vi "CANOpen_SetGet NMT Settings.vi"(6 "Set Parameters":bool, 8 "error in (no error)":errorcluster, 10 "Parameters":variant, 11 "NMT":T1={"Node run state"=128, "Emergency"=FALSE, "HB NG"={"Mode"=enum."None", "Update Time"=5, "Static detect in None"=enum."HB"}, "Delay for opp. state (ms)"=1000.0, "Node init static SDO state"=128, "Stop and Reset on Shutdown"=FALSE} {"Node init static SDO state" items=["start remote node"=1, "enter pre-operational"=128]; "Node run state" items=["start remote node"=1, "stop remote node"=2, "enter pre-operational"=128, "reset node"=129, "reset communication"=130]}) -> (0 "error out":errorcluster, 2 "Parameters":variant, 3 "NMT":T1={"Node run state"=128, "Emergency"=FALSE, "HB NG"={"Mode"=enum."None", "Update Time"=5, "Static detect in None"=enum."HB"}, "Delay for opp. state (ms)"=1000.0, "Node init static SDO state"=128, "Stop and Reset on Shutdown"=FALSE} {"Node init static SDO state" items=["start remote node"=1, "enter pre-operational"=128]; "Node run state" items=["start remote node"=1, "stop remote node"=2, "enter pre-operational"=128, "reset node"=129, "reset communication"=130]})   [LabVIEW 2021, in "CANOpen Addon Engine.lvlib"]
uses:
  CANOpen Addon Engine.lvlib
  CANOpen_NMT Settings.ctl
  Shared/CanOpen_NMT_Config.ctl
  Shared/CanOpen_NMT_Static detect.ctl
  Shared/CANOpen Addon GUID Lookup Global.vi
  Shared/CANOpen Addon Shared.lvlib
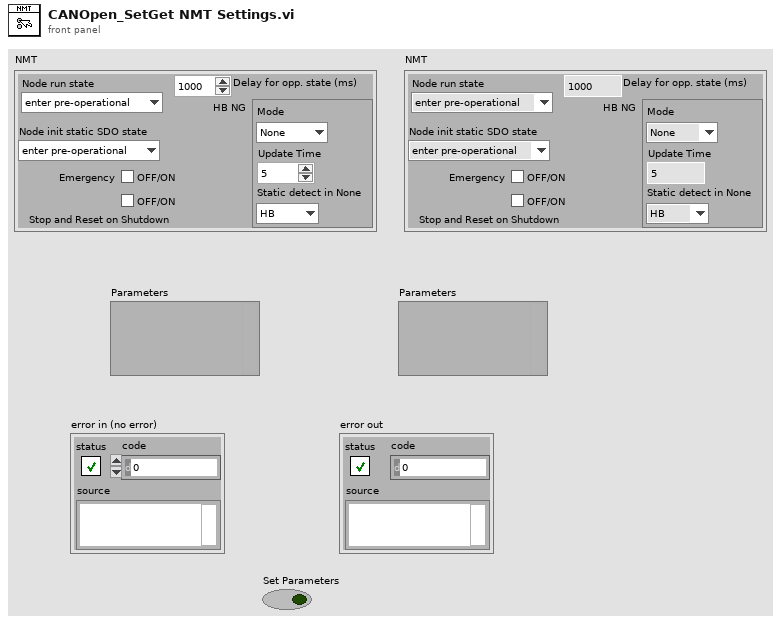
[diagram p1: front panel]
types:
  T1 = typedef "CANOpen Addon Engine.lvlib/CANOpen_NMT Settings.ctl" = cluster{"Node run state":u16, "Emergency":bool, "HB NG":T2, "Delay for opp. state (ms)":dbl, "Node init static SDO state":u16, "Stop and Reset on Shutdown":bool}
  T2 = typedef "CANOpen Addon Shared.lvlib/CanOpen_NMT_Config.ctl" = cluster{"Mode":T3, "Update Time":u16, "Static detect in None":T3}
  T3 = typedef "CANOpen Addon Shared.lvlib/CanOpen_NMT_Static detect.ctl" = enum16{"None", "HB", "NG"}
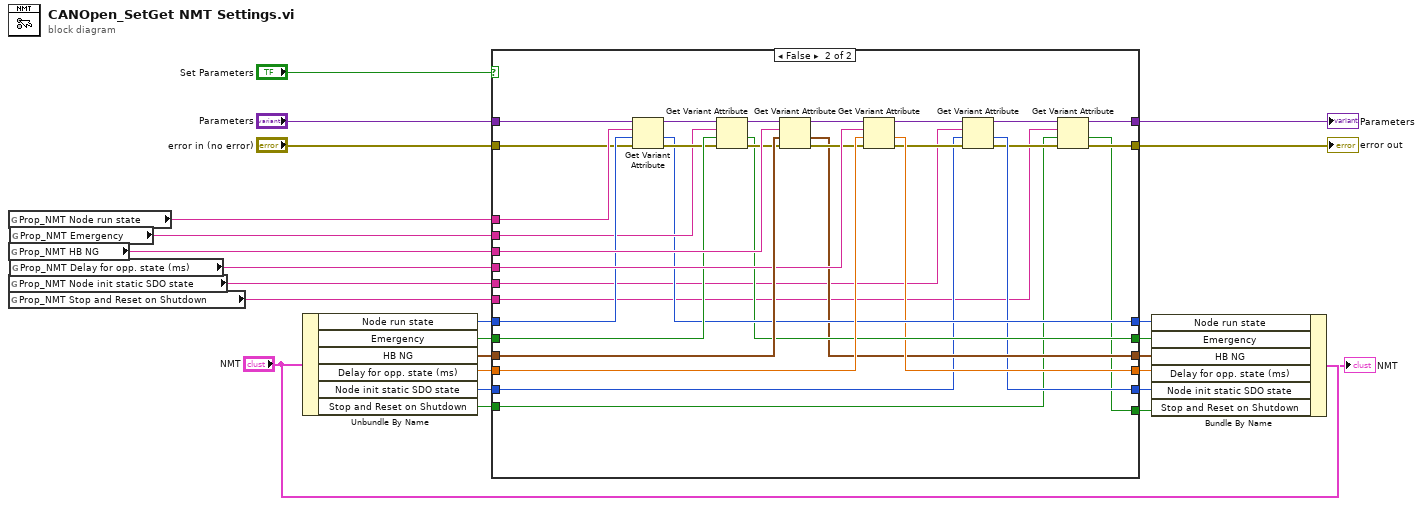
[diagram p0: block diagram]
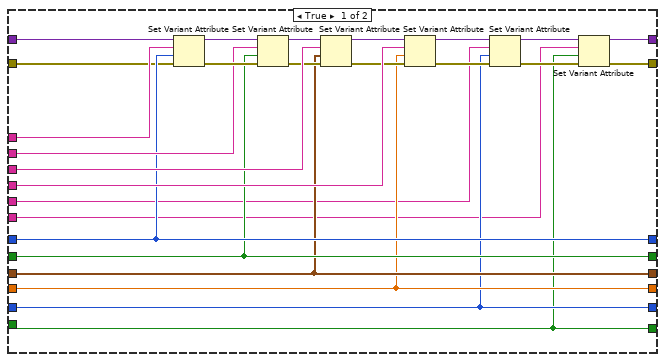
[diagram p2: hidden frame]
diagram:
  n1 = global read "CANOpen Addon GUID Lookup Global.vi" "Prop_NMT Node run state"() -> (w1:string)
  n2 = global read "CANOpen Addon GUID Lookup Global.vi" "Prop_NMT HB NG"() -> (w3:string)
  n3 = global read "CANOpen Addon GUID Lookup Global.vi" "Prop_NMT Node init static SDO state"() -> (w5:string)
  n4 = global read "CANOpen Addon GUID Lookup Global.vi" "Prop_NMT Stop and Reset on Shutdown"() -> (w6:string)
  n5 = global read "CANOpen Addon GUID Lookup Global.vi" "Prop_NMT Emergency"() -> (w2:string)
  n6 = global read "CANOpen Addon GUID Lookup Global.vi" "Prop_NMT Delay for opp. state (ms)"() -> (w4:string)
  n7 = Unbundle By Name("NMT") -> ("Node run state"=w18:u16, "Emergency"=w17:bool, "HB NG"=w16:T2, "Delay for opp. state (ms)"=w15:dbl, "Node init static SDO state"=w14:u16, "Stop and Reset on Shutdown"=w13:bool)
  n8 = case shown="False" "Set Parameters" {
    tunnel: [w30 w60] -> w25
    tunnel: [w31 w59] -> w24
    tunnel: w15 -> [w38 w83]
    tunnel: w16 -> [w39 w82]
    tunnel: w4 -> [w51 w81]
    tunnel: w3 -> [w50 w80]
    tunnel: w17 -> [w40 w75]
    tunnel: w18 -> [w41 w74]
    tunnel: "error in (no error)" -> [w27 w53]
    tunnel: w2 -> [w44 w72]
    tunnel: w1 -> [w42 w70]
    tunnel: "Parameters" -> [w26 w52]
    tunnel: [w41 w69] -> w12
    tunnel: [w40 w68] -> w11
    tunnel: [w38 w67] -> w9
    tunnel: [w39 w66] -> w10
    tunnel: w5 -> [w35 w62]
    tunnel: w14 -> [w34 w63]
    tunnel: [w34 w61] -> w8
    tunnel: w13 -> [w29 w56]
    tunnel: [w29 w55] -> w7
    tunnel: w6 -> [w28 w57]
    frame True {
      n9 = Set Variant Attribute(Variant=w26, name=w42, value=w41, error in=w27) -> (Variant out=w43:variant, error out=w45:errorcluster)  [unwired: 1 out]
      n10 = Set Variant Attribute(Variant=w43, name=w44, value=w40, error in=w45) -> (Variant out=w48:variant, error out=w49:errorcluster)  [unwired: 1 out]
      n11 = Set Variant Attribute(Variant=w48, name=w50, value=w39, error in=w49) -> (Variant out=w47:variant, error out=w46:errorcluster)  [unwired: 1 out]
      n12 = Set Variant Attribute(Variant=w47, name=w51, value=w38, error in=w46) -> (Variant out=w37:variant, error out=w36:errorcluster)  [unwired: 1 out]
      n13 = Set Variant Attribute(Variant=w37, name=w35, value=w34, error in=w36) -> (Variant out=w33:variant, error out=w32:errorcluster)  [unwired: 1 out]
      n14 = Set Variant Attribute(Variant=w33, name=w28, value=w29, error in=w32) -> (Variant out=w30:variant, error out=w31:errorcluster)  [unwired: 1 out]
    }
    frame False {
      n15 = Get Variant Attribute(Variant=w52, name=w70, default value (empty Variant)=w74, error in=w53) -> (duplicate Variant=w71:variant, value=w69:u16, error out=w73:errorcluster)  [unwired: 1 out]
      n16 = Get Variant Attribute(Variant=w71, name=w72, default value (empty Variant)=w75, error in=w73) -> (duplicate Variant=w78:variant, value=w68:bool, error out=w79:errorcluster)  [unwired: 1 out]
      n17 = Get Variant Attribute(Variant=w78, name=w80, default value (empty Variant)=w82, error in=w79) -> (duplicate Variant=w77:variant, value=w66:T2, error out=w76:errorcluster)  [unwired: 1 out]
      n18 = Get Variant Attribute(Variant=w77, name=w81, default value (empty Variant)=w83, error in=w76) -> (duplicate Variant=w64:variant, value=w67:dbl, error out=w65:errorcluster)  [unwired: 1 out]
      n19 = Get Variant Attribute(Variant=w64, name=w62, default value (empty Variant)=w63, error in=w65) -> (duplicate Variant=w54:variant, value=w61:u16, error out=w58:errorcluster)  [unwired: 1 out]
      n20 = Get Variant Attribute(Variant=w54, name=w57, default value (empty Variant)=w56, error in=w58) -> (duplicate Variant=w60:variant, value=w55:bool, error out=w59:errorcluster)  [unwired: 1 out]
    }
  }
  "Parameters" <- w25
  "error out" <- w24
  n21 = Bundle By Name(cluster="NMT", "Node run state"=w12, "Emergency"=w11, "HB NG"=w10, "Delay for opp. state (ms)"=w9, "Node init static SDO state"=w8, "Stop and Reset on Shutdown"=w7) -> (→"NMT":T1)
